vi "Init Device.vi"(8 "error in (no error)":errorcluster, 11 "cetoni in":refnum<class "cetoni.lvclass">) -> (0 "error out":errorcluster, 3 "cetoni out":refnum<class "cetoni.lvclass">)   [LabVIEW 2018, in "cetoni.lvlib" / "cetoni.lvclass"]
uses:
  cetoni.lvclass
  Device/Device.lvclass
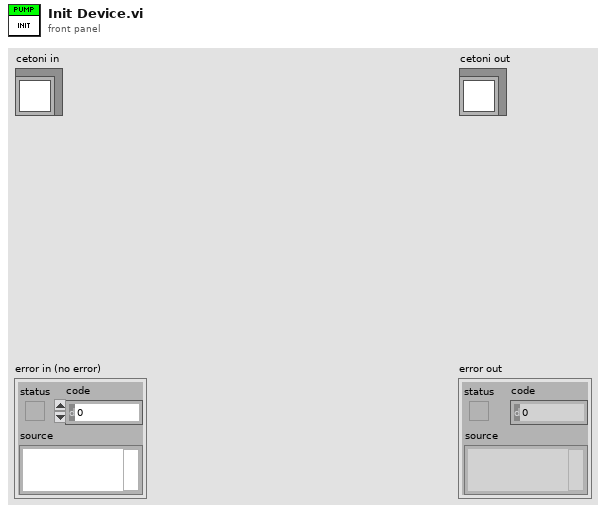
[diagram p1: front panel]
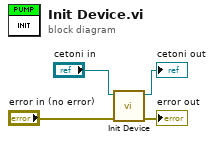
[diagram p0: block diagram]
diagram:
  n1 = call-parent "Init Device.vi"("error in (no error)"="error in (no error)", "Device in"="cetoni in") -> ("error out"=→"error out":errorcluster, "Device out"=→"cetoni out":refnum<class "cetoni.lvclass">)  [unwired: 8 in]
